vi "Read_calibration_files.vi"() -> ()   [LabVIEW 2010]
uses:
  Controls/Pressure_Units.ctl
  Controls/Post_Process.ctl
  Controls/Instrument_Array.ctl
  Globals/Meas_global.vi
  Acquisition/PWA/PWAtasksGLOBAL.vi
  Globals/Trav_pos_global.vi
panel:
  in  "Pressure Units":T1
  # "This Program Read data in from the calibration files"
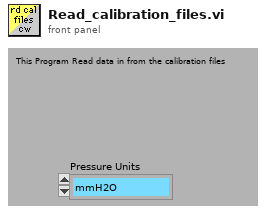
[diagram p1: front panel]
types:
  T1 = typedef "Pressure_Units.ctl" = enum16{"mmH2O", "mmHg", "Pa (N/m^2)", "mbar", "bar"}
  T2 = typedef "Analysis_info_cluster.ctl" = cluster{"Colour":u32, "Inst type":T3, "Inst name":string, "Symbol":string, "Code name":string, "Extra Info":string, "Inst Array":T4, "Index":i32, "Voltage Index":i32, "Extra Titles":string[], "Extra Values":string[]}
  T3 = typedef "Inst_type.ctl" = enum16{"Propeller anemometer", "Raw voltage", "Pressure Transducer", "Pitot-static tube", "Preston tube", "Hot wire", "Cross wire 1", "Cross wire 2", "Generic Linear", "Generic Polynomial", "Generic BackPoly", "Fast FID", "Thermocouple", "Cold wire", "Pulsed Wire", "LDA Vel", "LDA Tran time", "LDA Arr time"}
  T4 = typedef "Instrument_Array.ctl" = enum16{"PWA", "LDA", "Analogue"}
  T5 = typedef "PWA_Data.ctl" = enum16{"No PWA Data", "One Ch PWA"}
  T6 = typedef "Post_Process.ctl" = enum16{"Take New Data", "Post Process Raw Data File"}
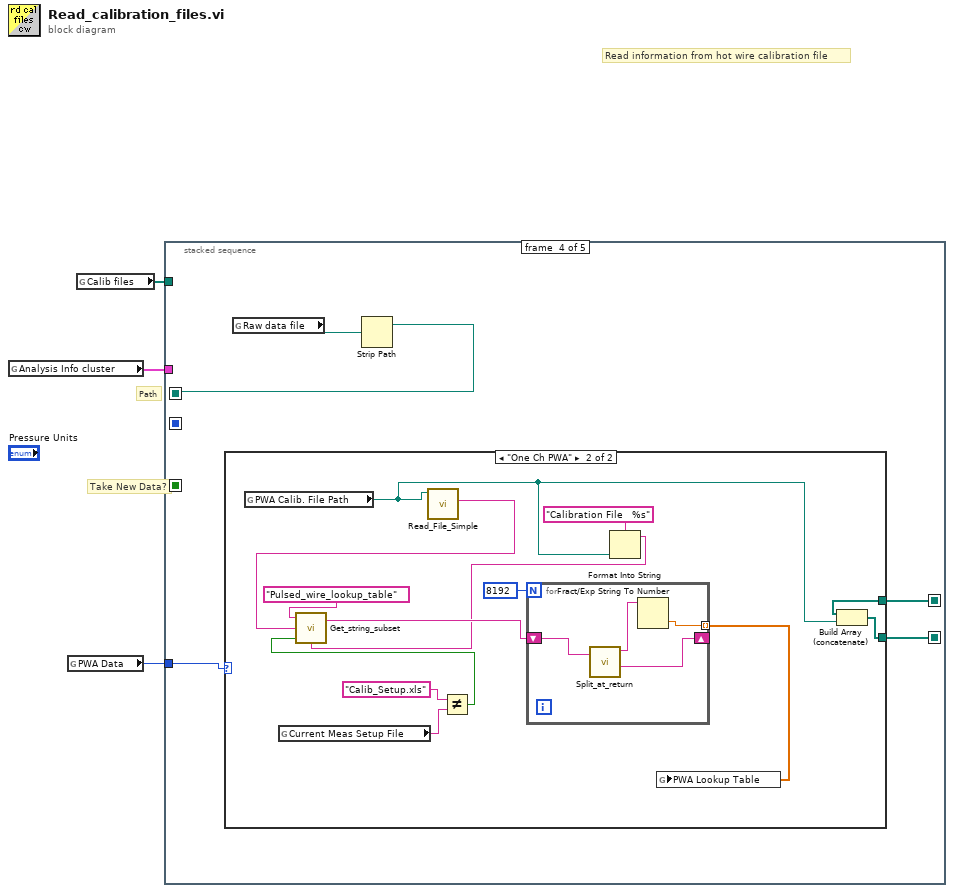
[diagram p0: block diagram]
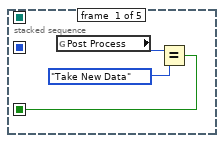
[diagram p2: hidden frame]
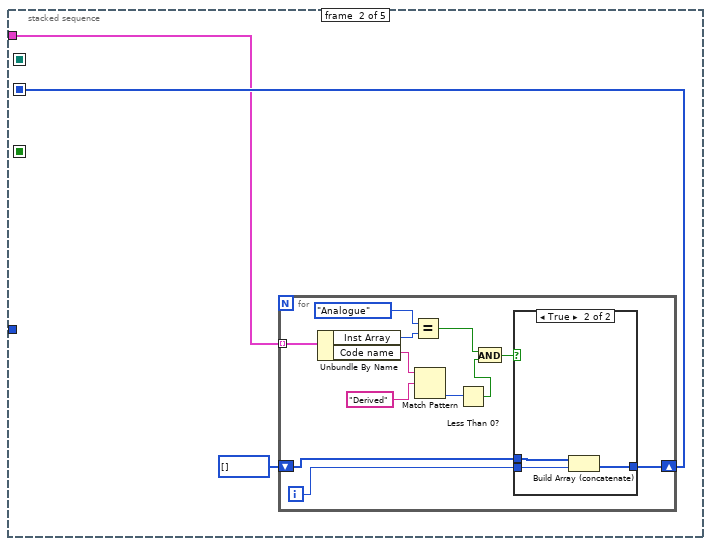
[diagram p3: hidden frame]
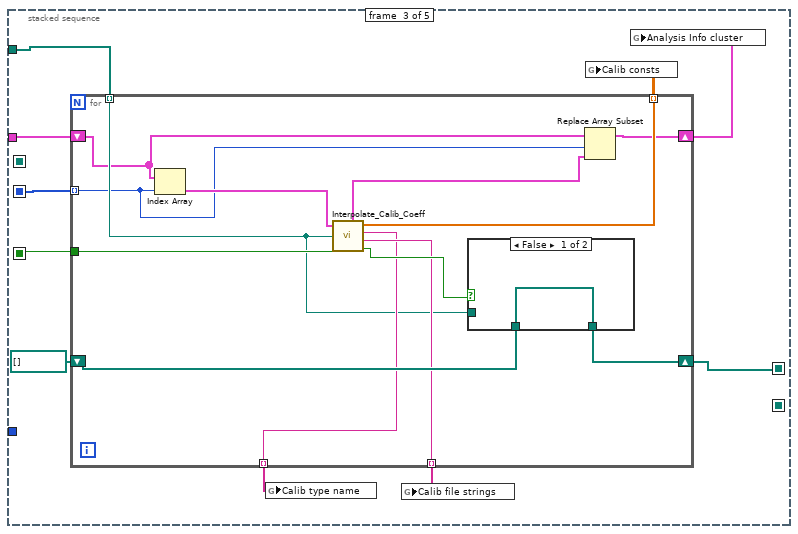
[diagram p5: hidden frame]
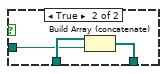
[diagram p6: hidden frame]
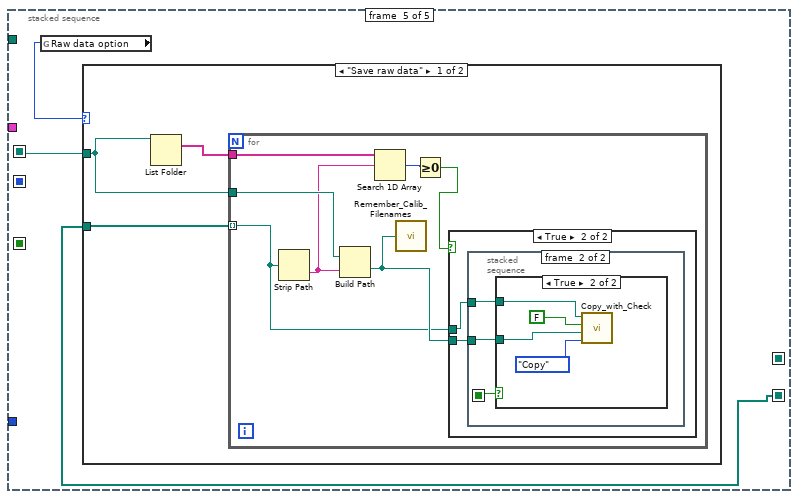
[diagram p8: hidden frame]
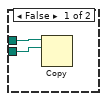
[diagram p9: hidden frame]
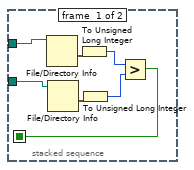
[diagram p10: hidden frame]
diagram:
  # "Take New Data?"
  # "Path"
  # "Read information from hot wire calibration file"
  n1 = global read "Meas_global.vi" "Analysis Info cluster"() -> (w1:T2[])
  n2 = global read "Meas_global.vi" "PWA Data"() -> (w2:T5)
  n3 = global read "Meas_global.vi" "Calib files"() -> (w3:path[])
  n4 = stacked-sequence {
    seq-local: [_ _ w35 _ _] -> [_ _ _ w53 _]
    seq-local: [_ _ _ w56 _] -> [_ _ _ _ w77]
    seq-local: [w4 _ _ _ _] -> [_ _ w33 _ _]
    seq-local: [_ _ _ w54 _] -> [_ _ _ _ w76]
    seq-local: [_ w8 _ _ _] -> [_ _ w27 _ _]
    tunnel: w3 -> [_ _ w32 _ _]
    tunnel: w2 -> [_ _ _ w55 _]
    tunnel: w1 -> [_ w7 w28 _ _]
    frame #0 {
      n5 = global read "Meas_global.vi" "Post Process"() -> (w5:T6)
      n6 = Equal?(x=w5, y=Post_Process."Take New Data" ("Post Process")) -> (x = y?=w4:bool)
    }
    frame #1 {
      n7 = for {
        tunnel: w7 -> [w13] mode=indexing
        shift-right: [w10] -> w8
        shift-left: i32[] [] -> [w11]
        i -> [w12]
        n8 = Unbundle By Name(w13) -> ("Inst Array"=w21:T4, "Code name"=w19:string)
        n9 = Equal?(x=Instrument_Array."Analogue" ("Inst Array"), y=w21) -> (x = y?=w15:bool)
        n10 = Match Pattern(string=w19, regular expression="Derived") -> (offset past match=w17:i32)  [unwired: 4 out]
        n11 = Less Than 0?(x=w17) -> (x < 0?=w16:bool)
        n12 = And(x=w15, y=w16) -> (x .and. y?=w14:bool)
        n13 = case shown="True" w14 {
          tunnel: w12 -> [_ w25]
          tunnel: w11 -> [w22 w24]
          tunnel: [w22 w23] -> w10
          frame False {
          }
          frame True {
            n14 = Build Array (concatenate)(w24, w25) -> (w23:i32[])
          }
        }
      }
    }
    frame #2 {
      n15 = for {
        tunnel: w32 -> [w41] mode=indexing
        shift-right: [w47] -> w35
        shift-left: path[] [] -> [w48]
        tunnel: w33 -> [w46]
        tunnel: [w44] -> w31 mode=indexing
        tunnel: [w43] -> w30 mode=indexing
        tunnel: [w42] -> w29 mode=indexing
        shift-right: [w37] -> w26
        shift-left: w28 -> [w39]
        tunnel: w27 -> [w38] mode=indexing
        n16 = Index Array(array=w39, index=w38) -> (element=w40:T2)
        n17 = call "Interpolate_Calib_Coeff.vi"("Analysis Info cluster"=w40, "Calib file"=w41, "Take New Data?"=w46) -> ("Calib Coeff"=w42:dbl[], "Calib Type Name"=w43:string, "Calib file string"=w44:string, "Read file"=w45:bool, "Analysis Info cluster  Out"=w36:T2)
        n18 = case shown="False" w45 {
          tunnel: w48 -> [w49 w52]
          tunnel: [w49 w51] -> w47
          tunnel: w41 -> [_ w50]
          frame False {
          }
          frame True {
            n19 = Build Array (concatenate)(w52, w50) -> (w51:path[])
          }
        }
        n20 = Replace Array Subset(array=w39, new element=w36, index=w38) -> (w37:T2[])
      }
      n21 = global write "Meas_global.vi" "Calib type name"(w30) -> ()
      n22 = global write "Meas_global.vi" "Calib file strings"(w31) -> ()
      n23 = global write "Meas_global.vi" "Calib consts"(w29) -> ()
      n24 = global write "Meas_global.vi" "Analysis Info cluster"(w26) -> ()
    }
    frame #3 {
      n25 = case shown="\"One Ch PWA\"" w55 {
        tunnel: [w58 w62] -> w54
        tunnel: w53 -> [w58 w63]
        frame "No PWA Data" {
        }
        frame "One Ch PWA" {
          n26 = global read "PWAtasksGLOBAL.vi" "PWA Calib. File Path"() -> (w60:path)
          n27 = global read "Trav_pos_global.vi" "Current Meas Setup File"() -> (w70:string)
          n28 = call "Read_File_Simple.vi"("Filename"=w60) -> ("string"=w64:string)  [unwired: 2 in, 7 out]
          n29 = Not Equal?(x="Calib_Setup.xls", y=w70) -> (x != y?=w71:bool)
          n30 = Format Into String(format string="Calibration File   %s", w60) -> (resulting string=w59:string)  [unwired: 2 in, 1 out]
          n31 = call "Get_string_subset.vi"("String Name"=w59, "Show Dialog?"=w71, "String to split"=w64, "File Label"="Pulsed_wire_lookup_table") -> ("Output string"=w66:string)  [unwired: 1 out]
          n32 = for {
            N: 8192 -> [_]
            shift-right: [w74] -> _
            shift-left: w66 -> [w75]
            tunnel: [w72] -> w67 mode=indexing
            n33 = call "Split_at_return.vi"("String"=w75) -> ("before substring"=w73:string, "after substring"=w74:string)  [unwired: 1 in, 2 out]
            n34 = Fract/Exp String To Number(string=w73) -> (number=w72:dbl)  [unwired: 4 out]
          }
          n35 = global write "PWAtasksGLOBAL.vi" "PWA Lookup Table"(w67) -> ()
          n36 = Build Array (concatenate)(w63, w60) -> (w62:path[])
        }
      }
      n37 = global read "Meas_global.vi" "Raw data file"() -> (w57:path)
      n38 = Strip Path(path=w57) -> (stripped path=w56:path)  [unwired: 1 out]
    }
    frame #4 {
      n39 = global read "Meas_global.vi" "Raw data option"() -> (w78:enum16{"Save raw data", "Raw data not saved"})
      n40 = case shown="\"Save raw data\"" w78 {
        tunnel: w76 -> [w81 _]
        tunnel: w77 -> [w79 _]
        frame "Save raw data" {
          n41 = List Folder(path=w79) -> (filenames=w80:string[])  [unwired: 1 in, 5 out]
          n42 = for {
            tunnel: w81 -> [w82] mode=indexing
            tunnel: w79 -> [w85]
            tunnel: w80 -> [w88]
            n43 = Strip Path(path=w82) -> (name=w84:string)  [unwired: 1 out]
            n44 = Build Path(base path=w85, name or relative path=w84) -> (appended path=w83:path)
            n45 = Search 1D Array(1D array=w88, element=w84) -> (index of element=w87:i32)  [unwired: 1 out]
            n46 = call "Remember_Calib_Filenames.vi"("Filename to Remember"=w83) -> ()  [unwired: 1 out]
            n47 = Greater Or Equal To 0?(x=w87) -> (x >= 0?=w86:bool)
            n48 = case shown="True" w86 {
              tunnel: w83 -> [w90 w91]
              tunnel: w82 -> [w89 w92]
              frame False {
                n49 = Copy(10:w90, 11:w89) -> ()  [unwired: 1 in, 5 out]
              }
              frame True {
                n50 = stacked-sequence {
                  seq-local: [w95 _] -> [_ w102]
                  tunnel: w92 -> [w99 w100]
                  tunnel: w91 -> [w98 w101]
                  frame #0 {
                    n51 = File/Directory Info(path=w99) -> (last mod=w93:timestamp)  [unwired: 1 in, 6 out]
                    n52 = File/Directory Info(path=w98) -> (last mod=w94:timestamp)  [unwired: 1 in, 6 out]
                    n53 = To Unsigned Long Integer(number=w93) -> (unsigned 32bit integer=w97:u32)
                    n54 = To Unsigned Long Integer(number=w94) -> (unsigned 32bit integer=w96:u32)
                    n55 = Greater?(x=w97, y=w96) -> (0:w95:bool)
                  }
                  frame #1 {
                    n56 = case shown="True" w102 {
                      tunnel: w101 -> [_ w105]
                      tunnel: w100 -> [_ w106]
                      frame False {
                      }
                      frame True {
                        n57 = call "Copy_with_Check.vi"("Mode"=enum16{"Move", "Copy"}."Copy", "Target Path"=w105, "Variable Target?"=FALSE, "Source Path"=w106) -> ()  [unwired: 1 out]
                      }
                    }
                  }
                }
              }
            }
          }
        }
        frame "Raw data not saved" {
        }
      }
    }
  }
